vi "IMMU - Convert Accelerometer.vi"(9 "Accel Offset Array In":i16[](array[numeric]), 11 "Input Raw Accel Array (U8)":u8[](array[numeric])) -> (3 "Output Acceleration Array (ms^2)":dbl[](array[numeric]))   [LabVIEW 2021]
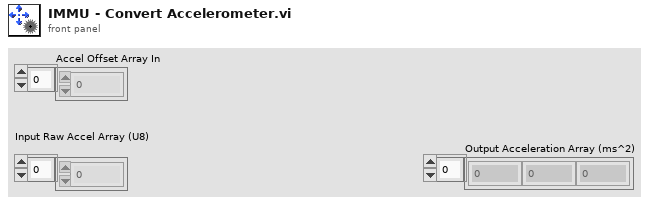
[diagram p1: front panel]
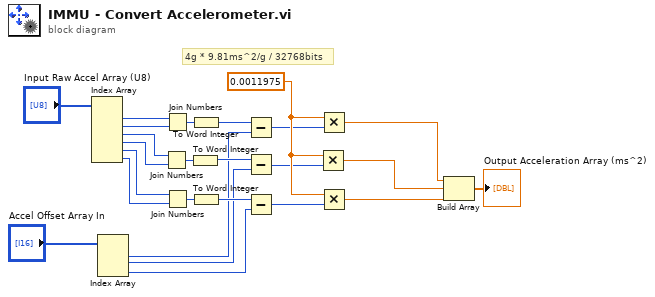
[diagram p0: block diagram]
diagram:
  w12 = 0.0011975 ("y")
  # "4g * 9.81ms^2/g / 32768bits"
  n1 = Index Array(array="Input Raw Accel Array (U8)") -> (element #1=w24:u8, element #2=w25:u8, element #3=w18:u8, element #4=w17:u8, element #5=w16:u8, element #6=w15:u8)  [unwired: 6 in]
  n2 = Index Array(array="Accel Offset Array In") -> (element #1=w3:i16, element #2=w2:i16, element #3=w1:i16)  [unwired: 3 in]
  n3 = Join Numbers(hi=w18, lo=w17) -> ((hi.lo)=w20:u16)
  n4 = Join Numbers(hi=w24, lo=w25) -> ((hi.lo)=w22:u16)
  n5 = Join Numbers(hi=w16, lo=w15) -> ((hi.lo)=w19:u16)
  n6 = To Word Integer(number=w20) -> (16bit integer=w5:i16)
  n7 = To Word Integer(number=w22) -> (16bit integer=w9:i16)
  n8 = To Word Integer(number=w19) -> (16bit integer=w4:i16)
  n9 = Subtract(x=w9, y=w3) -> (x-y=w8:i16)
  n10 = Subtract(x=w5, y=w2) -> (x-y=w6:i16)
  n11 = Subtract(x=w4, y=w1) -> (x-y=w7:i16)
  n12 = Multiply(x=w12, y=w6) -> (x*y=w13:dbl)
  n13 = Multiply(x=w12, y=w8) -> (x*y=w21:dbl)
  n14 = Multiply(x=w12, y=w7) -> (x*y=w14:dbl)
  n15 = Build Array(w21, w13, w14) -> (→"Output Acceleration Array (ms^2)":dbl[])
